vi "Check position.vi"(8 "error in (no error)":errorcluster, 11 "StageSPIM in":refnum<class "StageSPIM.lvclass">) -> (0 "error out":errorcluster, 3 "StageSPIM out":refnum<class "StageSPIM.lvclass">)   [LabVIEW 2012, in "StageSPIM.lvclass"]
uses:
  StageSPIM.lvclass
  <vilib>/Distrio/Murmex/ProceedMessage/ProceedMessage.lvclass
  <vilib>/Distrio/Murmex/GenericMessage/GenericMessage.lvclass
  StageSPIM.lvclass/StageSPIM.ctl
  <vilib>/Distrio/Murmex/Message/Add or replace parameter.vi
  <vilib>/Distrio/Murmex/Murmex/Murmex.lvclass
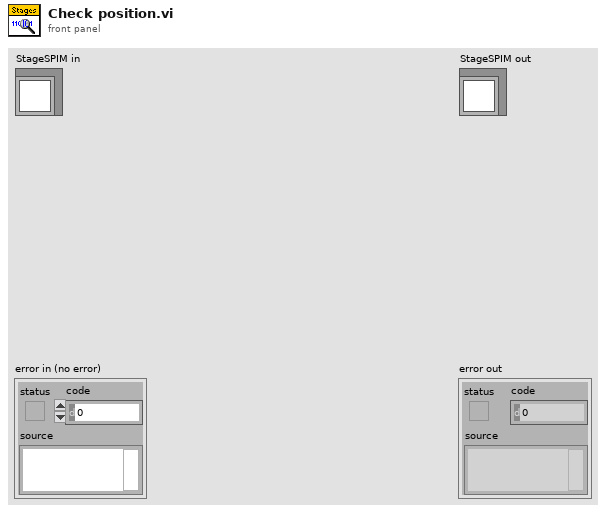
[diagram p1: front panel]
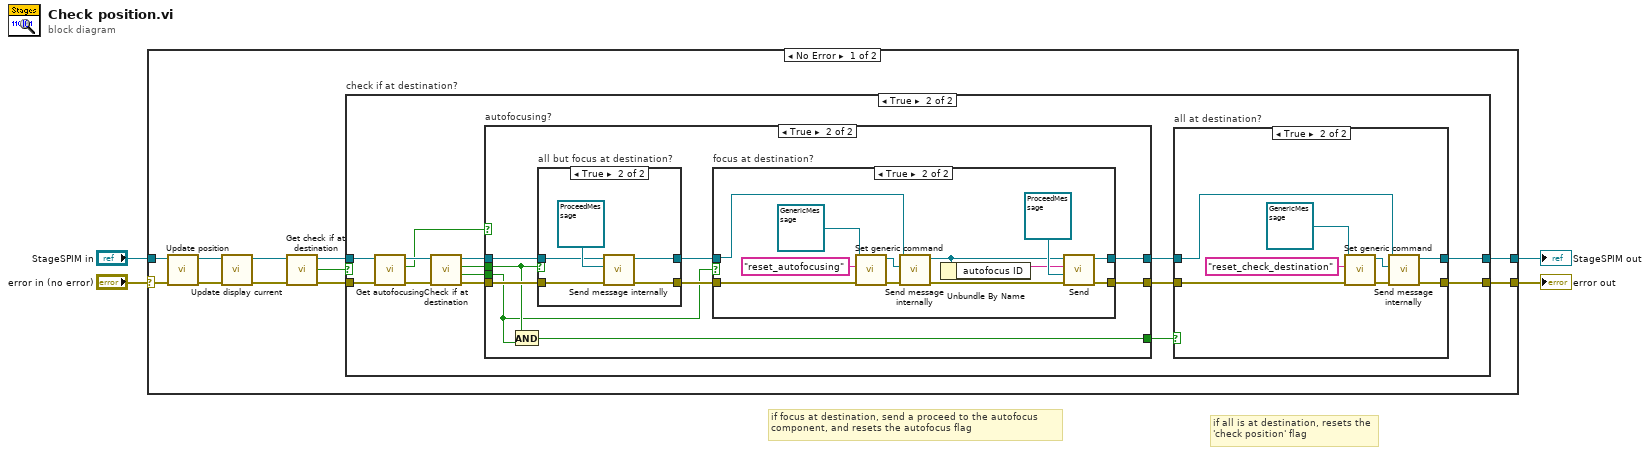
[diagram p0: block diagram]
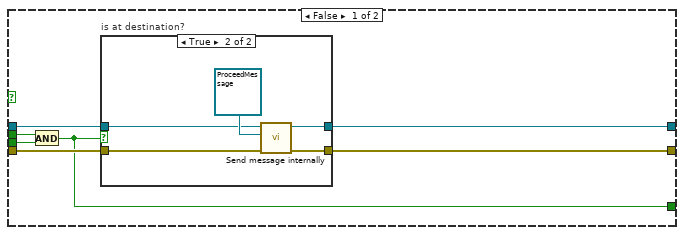
[diagram p4: hidden frame]
diagram:
  # "if all is at destination, resets the\n'check position' flag"
  # "if focus at destination, send a proceed to the autofocus\ncomponent, and resets the autofocus flag"
  n1 = case shown="No Error" "error in (no error)" {
    selector: "error in (no error)" -> [w8 w87]
    tunnel: [w7 w87] -> w3
    tunnel: [w5 w86] -> w1
    tunnel: "StageSPIM in" -> [w6 w86]
    frame No Error {
      n2 = call-dynamic "Update position.vi"("error in (no error)"=w8, "StageSPIM in"=w6) -> ("error out"=w12:errorcluster, "StageSPIM out"=w10:refnum<class "StageSPIM.lvclass">)  [unwired: 8 in]
      n3 = call-dynamic "Update display current.vi"("error in (no error)"=w12, "StageSPIM in"=w10) -> ("error out"=w11:errorcluster, "StageSPIM out"=w9:refnum<class "StageSPIM.lvclass">)  [unwired: 8 in]
      n4 = call-dynamic "Get check if at destination.vi"("error in (no error)"=w11, "StageSPIM in"=w9) -> ("error out"=w14:errorcluster, "check if at destination"=w15:bool, "StageSPIM out"=w13:refnum<class "StageSPIM.lvclass">)  [unwired: 7 in]
      n5 = case "check if at destination?" shown="True" w15 {
        tunnel: w14 -> [w17 w28]
        tunnel: w13 -> [w16 w26]
        tunnel: [w16 w20] -> w5
        tunnel: [w17 w19] -> w7
        frame False {
        }
        frame True {
          n6 = call-dynamic "Get autofocusing.vi"("error in (no error)"=w28, "StageSPIM in"=w26) -> ("error out"=w27:errorcluster, "autofocusing?"=w24:bool, "StageSPIM out"=w25:refnum<class "StageSPIM.lvclass">)  [unwired: 7 in]
          n7 = call-dynamic "Check if at destination.vi"("error in (no error)"=w27, "StageSPIM in"=w25) -> ("error out"=w30:errorcluster, "focus at destination?"=w23:bool, "at destination? (all but focus)"=w31:bool, "StageSPIM out"=w29:refnum<class "StageSPIM.lvclass">)  [unwired: 6 in]
          n8 = case "autofocusing?" shown="True" w24 {
            tunnel: w31 -> [w44 w60]
            tunnel: w30 -> [w48 w64]
            tunnel: w29 -> [w47 w63]
            tunnel: [w46 w58] -> w22
            tunnel: [w45 w57] -> w21
            tunnel: w23 -> [w43 w59]
            tunnel: [w42 w56] -> w18
            frame False {
              n9 = And(x=w44, y=w43) -> (x .and. y?=w42:bool)
              n10 = case "is at destination?" shown="True" w42 {
                tunnel: w48 -> [w50 w51]
                tunnel: w47 -> [w49 w52]
                tunnel: [w50 w54] -> w45
                tunnel: [w49 w53] -> w46
                frame False {
                }
                frame True {
                  n11 = call <vilib>:"Send message internally.vi"("error in (no error)"=w51, "Message"=refnum<class "ProceedMessage.lvclass"> refnum ("Distrio Murmex 1.1:ProceedMessage"), "Murmex in"=w52) -> ("error out"=w54:errorcluster, "Murmex out"=w53:refnum<class "StageSPIM.lvclass">)  [unwired: 7 in]
                }
              }
            }
            frame True {
              n12 = And(x=w60, y=w59) -> (x .and. y?=w56:bool)
              n13 = case "all but focus at destination?" shown="True" w60 {
                tunnel: w64 -> [w80 w81]
                tunnel: w63 -> [w79 w82]
                tunnel: [w80 w84] -> w61
                tunnel: [w79 w83] -> w62
                frame False {
                }
                frame True {
                  n14 = call <vilib>:"Send message internally.vi"("error in (no error)"=w81, "Message"=refnum<class "ProceedMessage.lvclass"> refnum ("Distrio Murmex 1.1:ProceedMessage"), "Murmex in"=w82) -> ("error out"=w84:errorcluster, "Murmex out"=w83:refnum<class "StageSPIM.lvclass">)  [unwired: 7 in]
                }
              }
              n15 = case "focus at destination?" shown="True" w59 {
                tunnel: w61 -> [w66 w72]
                tunnel: w62 -> [w65 w69]
                tunnel: [w66 w75] -> w57
                tunnel: [w65 w76] -> w58
                frame False {
                }
                frame True {
                  n16 = call <vilib>:"Set generic command.vi"("error in (no error)"=w72, "generic command"="reset_autofocusing", "GenericMessage in"=refnum<class "GenericMessage.lvclass"> refnum ("Message in")) -> ("error out"=w73:errorcluster, "GenericMessage out"=w68:refnum<class "GenericMessage.lvclass">)  [unwired: 7 in]
                  n17 = call <vilib>:"Send message internally.vi"("error in (no error)"=w73, "Message"=w68, "Murmex in"=w69) -> ("error out"=w71:errorcluster, "Murmex out"=w70:refnum<class "StageSPIM.lvclass">)  [unwired: 7 in]
                  n18 = Unbundle By Name(w70) -> ("autofocus ID"=w77:string)
                  n19 = call <vilib>:"Send.vi"("error in (no error)"=w71, "Message"=refnum<class "ProceedMessage.lvclass"> refnum ("Distrio Murmex 1.1:ProceedMessage"), "recipient"=w77, "Murmex in"=w70) -> ("error out"=w75:errorcluster, "Murmex out"=w76:refnum<class "StageSPIM.lvclass">)  [unwired: 6 in]
                }
              }
            }
          }
          n20 = case "all at destination?" shown="True" w18 {
            tunnel: w22 -> [w33 w38]
            tunnel: w21 -> [w32 w36]
            tunnel: [w33 w37] -> w20
            tunnel: [w32 w34] -> w19
            frame False {
            }
            frame True {
              n21 = call <vilib>:"Set generic command.vi"("error in (no error)"=w36, "generic command"="reset_check_destination", "GenericMessage in"=refnum<class "GenericMessage.lvclass"> refnum ("Message in")) -> ("error out"=w35:errorcluster, "GenericMessage out"=w40:refnum<class "GenericMessage.lvclass">)  [unwired: 7 in]
              n22 = call <vilib>:"Send message internally.vi"("error in (no error)"=w35, "Message"=w40, "Murmex in"=w38) -> ("error out"=w34:errorcluster, "Murmex out"=w37:refnum<class "StageSPIM.lvclass">)  [unwired: 7 in]
            }
          }
        }
      }
    }
    frame Error {
    }
  }
  "error out" <- w3
  "StageSPIM out" <- w1
